vi "CFG Build Array Value.vi"(0 "Value String":string, 5 "Delimiter(s)":string, 7 "Dimensions":i32, 9 "Element Type":T1, 11 "error in":errorcluster, 13 "Float":bool) -> (4 "Variant":variant, 15 "error out":errorcluster)   [LabVIEW 2012]
uses:
  Type Defs/CFG Tag Type Enum.ctl
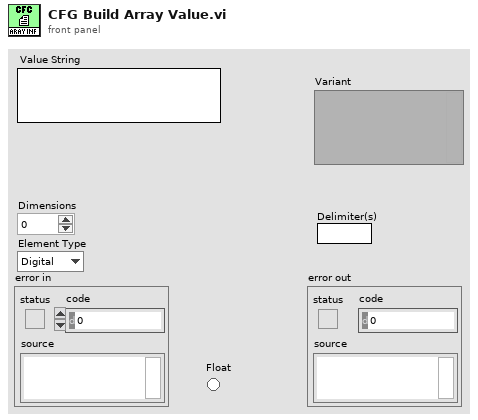
[diagram p1: front panel]
types:
  T1 = typedef "CFG Tag Type Enum.ctl" = enum16{"Digital", "Slide", "Enum", "Boolean", "String", "Path", "Array", "VISAResourceName", "DAQmxName", "Cluster"}
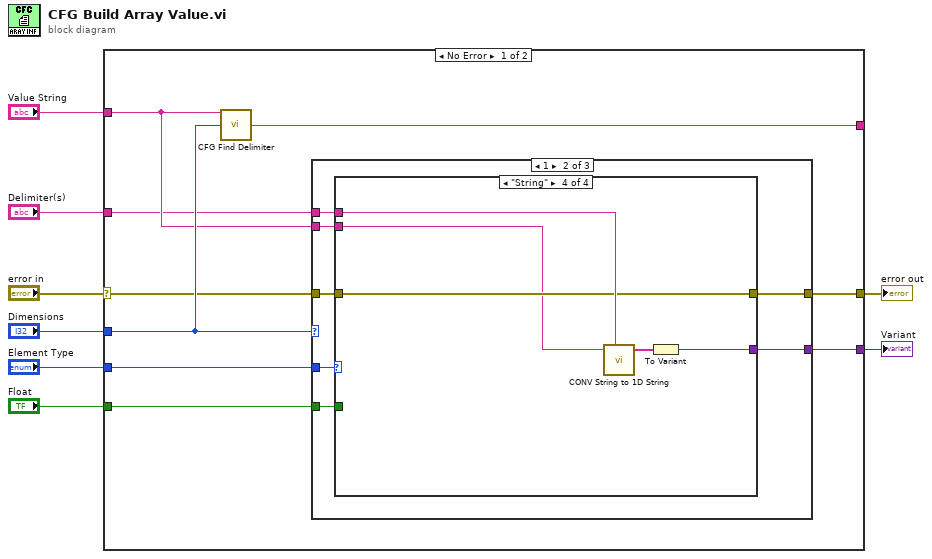
[diagram p0: block diagram]
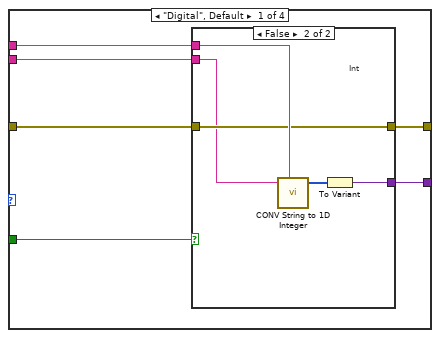
[diagram p3: hidden frame]
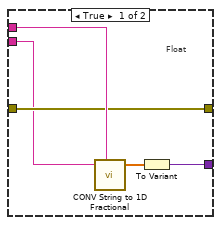
[diagram p4: hidden frame]
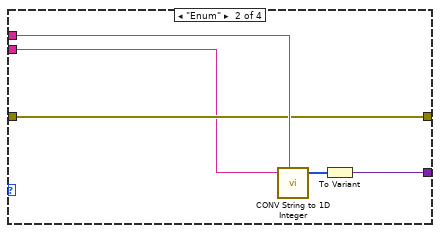
[diagram p5: hidden frame]
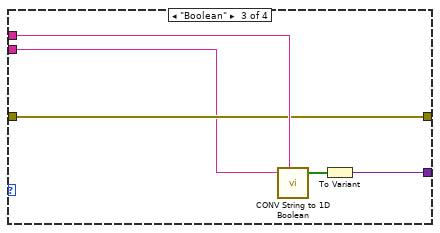
[diagram p6: hidden frame]
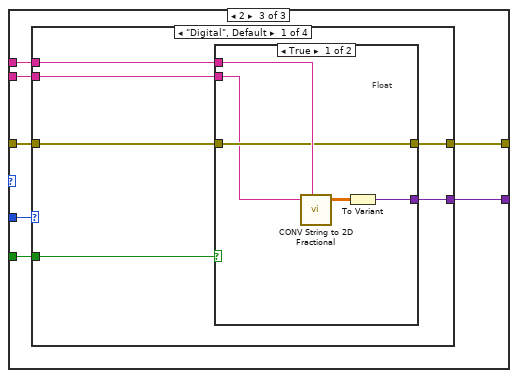
[diagram p7: hidden frame]
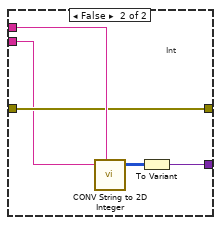
[diagram p8: hidden frame]
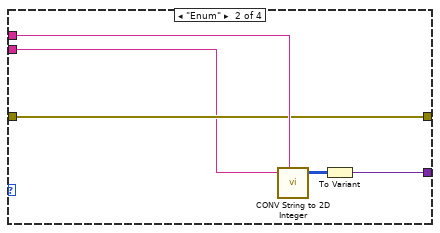
[diagram p9: hidden frame]
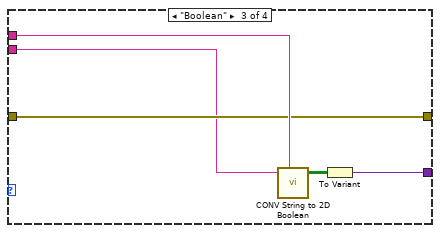
[diagram p10: hidden frame]
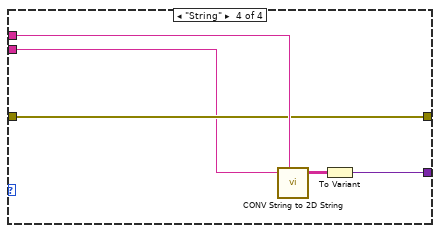
[diagram p11: hidden frame]
diagram:
  n1 = case shown="No Error" "error in" {
    selector: "error in" -> [w11 w95]
    tunnel: [w9 _] -> _
    tunnel: [w17 _] -> w2
    tunnel: [w16 w95] -> w8
    tunnel: "Value String" -> [w12 _]
    tunnel: "Dimensions" -> [w15 _]
    tunnel: "Element Type" -> [w14 _]
    tunnel: "Float" -> [w13 _]
    tunnel: "Delimiter(s)" -> [w10 _]
    frame No Error {
      n2 = call "CFG Find Delimiter.vi"("Value"=w12, "Dimensions"=w15) -> ("Delimiter (s)"=w9:string)  [unwired: 1 in, 12 out]
      n3 = case shown="1" w15 {
        tunnel: w14 -> [_ w25 w63]
        tunnel: w10 -> [_ w24 w62]
        tunnel: [_ w23 w61] -> w17
        tunnel: w12 -> [_ w22 w60]
        tunnel: [w18 w21 w59] -> w16
        tunnel: w11 -> [w18 w20 w58]
        tunnel: w13 -> [_ w19 w57]
        frame Default {
        }
        frame 1 {
          n4 = case shown="\"String\"" w25 {
            tunnel: w24 -> [w31 w46 w51 w56]
            tunnel: [w30 w45 w50 w55] -> w23
            tunnel: w22 -> [w28 w43 w48 w53]
            tunnel: [w29 w44 w49 w54] -> w21
            tunnel: w20 -> [w26 w44 w49 w54]
            tunnel: w19 -> [w27 _ _ _]
            frame "Digital", Default {
              n5 = case shown="False" w27 {
                tunnel: w31 -> [w36 w41]
                tunnel: [w32 w37] -> w30
                tunnel: w26 -> [w35 w40]
                tunnel: [w35 w40] -> w29
                tunnel: w28 -> [w34 w39]
                frame True {
                  # "Float"
                  n6 = call "CONV String to 1D Fractional.vi"("String"=w34, "Delimiter (,)"=w36) -> ("1-D Fractional"=w33:dbl[])  [unwired: 7 out]
                  n7 = To Variant(anything=w33) -> (Variant=w32:variant)
                }
                frame False {
                  # "Int"
                  n8 = call "CONV String to 1D Integer.vi"("String"=w39, "Delimiter (,)"=w41) -> ("1-D Integer"=w38:i32[])  [unwired: 7 out]
                  n9 = To Variant(anything=w38) -> (Variant=w37:variant)
                }
              }
            }
            frame "Enum" {
              n10 = call "CONV String to 1D Integer.vi"("String"=w43, "Delimiter (,)"=w46) -> ("1-D Integer"=w42:i32[])  [unwired: 7 out]
              n11 = To Variant(anything=w42) -> (Variant=w45:variant)
            }
            frame "Boolean" {
              n12 = call "CONV String to 1D Boolean.vi"("String"=w48, "Delimiter (,)"=w51) -> ("1-D Boolean"=w47:bool[])  [unwired: 7 out]
              n13 = To Variant(anything=w47) -> (Variant=w50:variant)
            }
            frame "String" {
              n14 = call "CONV String to 1D String.vi"("String"=w53, "Delimiter (,)"=w56) -> ("1-D String"=w52:string[])  [unwired: 7 out]
              n15 = To Variant(anything=w52) -> (Variant=w55:variant)
            }
          }
        }
        frame 2 {
          n16 = case shown="\"Digital\", Default" w63 {
            tunnel: w62 -> [w69 w84 w89 w94]
            tunnel: [w68 w83 w88 w93] -> w61
            tunnel: w60 -> [w66 w81 w86 w91]
            tunnel: [w67 w82 w87 w92] -> w59
            tunnel: w58 -> [w64 w82 w87 w92]
            tunnel: w57 -> [w65 _ _ _]
            frame "Digital", Default {
              n17 = case shown="True" w65 {
                tunnel: w69 -> [w74 w79]
                tunnel: [w70 w75] -> w68
                tunnel: w64 -> [w73 w78]
                tunnel: [w73 w78] -> w67
                tunnel: w66 -> [w72 w77]
                frame True {
                  # "Float"
                  n18 = call "CONV String to 2D Fractional.vi"("String"=w72, "Delimiters (,;)"=w74) -> ("2-D Fractional"=w71:dbl[][])  [unwired: 7 out]
                  n19 = To Variant(anything=w71) -> (Variant=w70:variant)
                }
                frame False {
                  # "Int"
                  n20 = call "CONV String to 2D Integer.vi"("String"=w77, "Delimiters (,;)"=w79) -> ("2-D Integer"=w76:i32[][])  [unwired: 7 out]
                  n21 = To Variant(anything=w76) -> (Variant=w75:variant)
                }
              }
            }
            frame "Enum" {
              n22 = call "CONV String to 2D Integer.vi"("String"=w81, "Delimiters (,;)"=w84) -> ("2-D Integer"=w80:i32[][])  [unwired: 7 out]
              n23 = To Variant(anything=w80) -> (Variant=w83:variant)
            }
            frame "Boolean" {
              n24 = call "CONV String to 2D Boolean.vi"("String"=w86, "Delimiters (,;)"=w89) -> ("2-D Boolean"=w85:bool[][])  [unwired: 7 out]
              n25 = To Variant(anything=w85) -> (Variant=w88:variant)
            }
            frame "String" {
              n26 = call "CONV String to 2D String.vi"("String"=w91, "Delimiters (,;)"=w94) -> ("2-D String"=w90:string[][])  [unwired: 7 out]
              n27 = To Variant(anything=w90) -> (Variant=w93:variant)
            }
          }
        }
      }
    }
    frame Error {
    }
  }
  "error out" <- w8
  "Variant" <- w2
